vi "NMEA_ParseMessage-WIMDA.vi"(9 "Error In":errorcluster, 10 "$WIMDA-message_IN":string="$WIMDA,29.7101,I,1.0061,B,28.7,C,,,60.8,,20.3,C,,,,,,,,*7B") -> (1 "Error Out":errorcluster, 2 "$WIMDA-message_OUT":T1)   [LabVIEW 2016, in "AIRMAR WeatherCaster.lvlib"]
doc: "<B>GPGGA</B>\nGlobal Positioning System Fix Data"
uses:
  AIRMAR WeatherCaster.lvlib
  NMEA_WIMDA-data.ctl
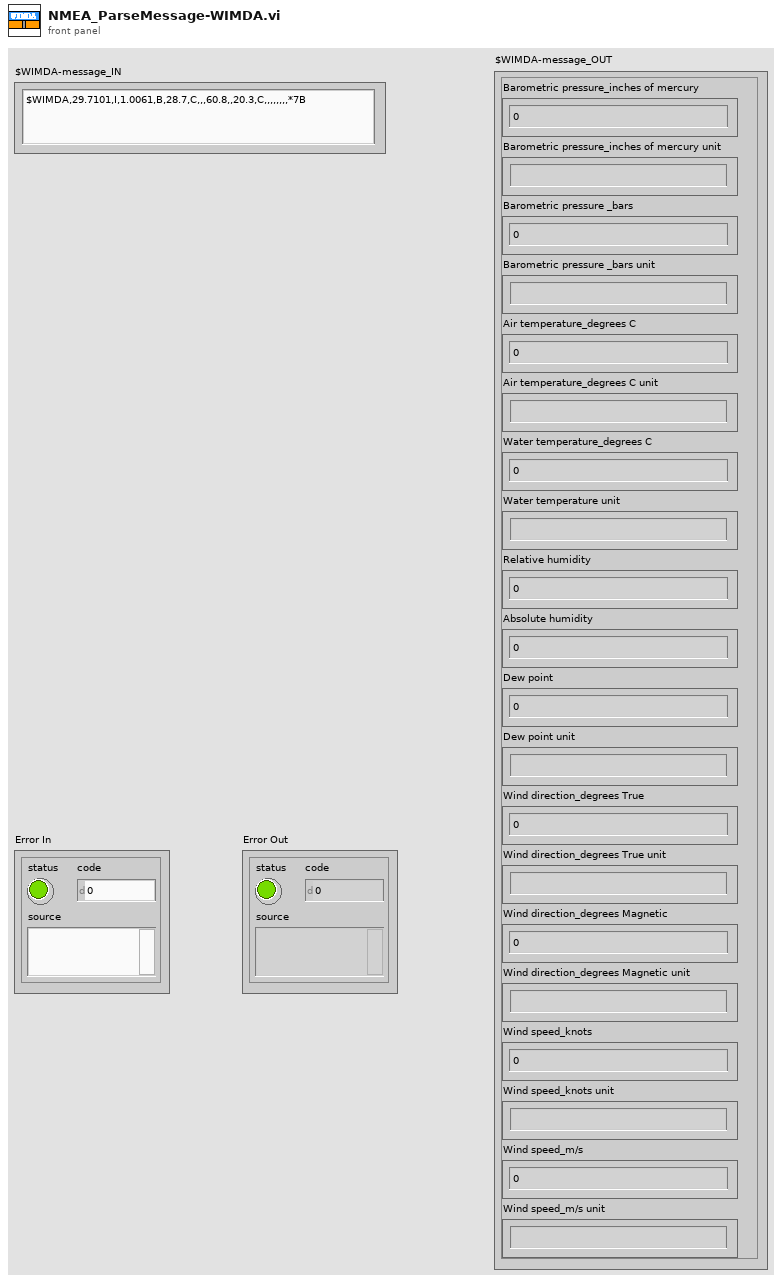
[diagram p1: front panel]
types:
  T1 = typedef "AIRMAR WeatherCaster.lvlib/NMEA_WIMDA-data.ctl" = cluster{"Barometric pressure_inches of mercury":dbl, "Barometric pressure_inches of mercury unit":string, "Barometric pressure _bars":dbl, "Barometric pressure _bars unit":string, "Air temperature_degrees C":dbl, "Air temperature_degrees C unit":string, "Water temperature_degrees C":dbl, "Water temperature unit":string, "Relative humidity":dbl, "Absolute humidity":dbl, "Dew point":dbl, "Dew point unit":string, "Wind direction_degrees True":dbl, "Wind direction_degrees True unit":string, "Wind direction_degrees Magnetic":dbl, "Wind direction_degrees Magnetic unit":string, "Wind speed_knots":dbl, "Wind speed_knots unit":string, "Wind speed_m/s":dbl, "Wind speed_m/s unit":string}
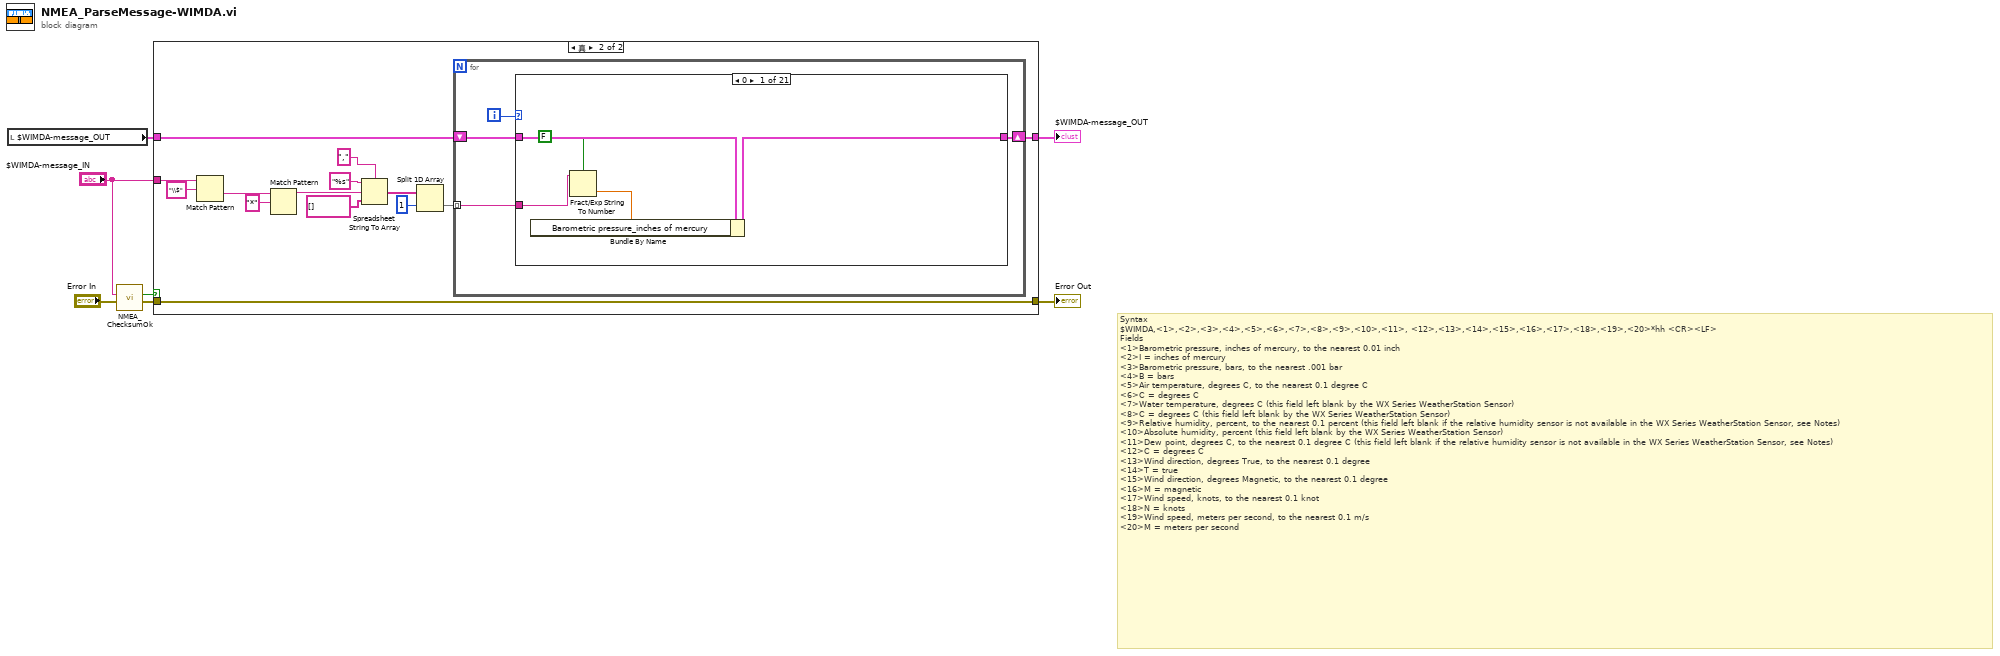
[diagram p0: block diagram]
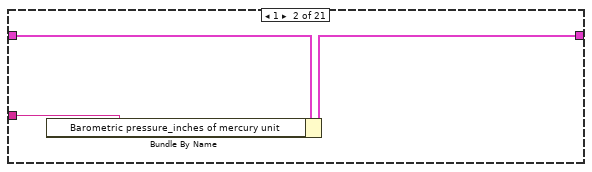
[diagram p3: hidden frame]
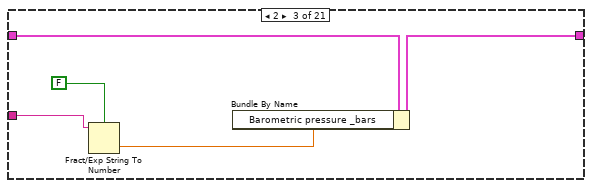
[diagram p4: hidden frame]
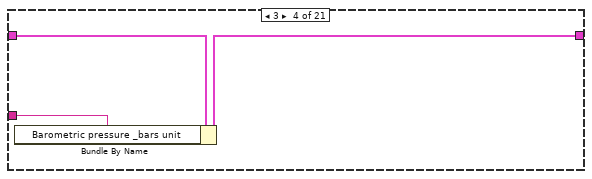
[diagram p5: hidden frame]
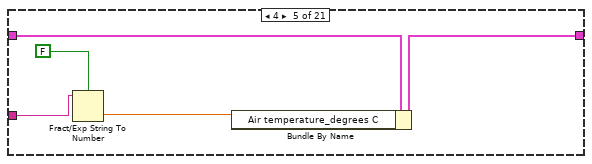
[diagram p6: hidden frame]
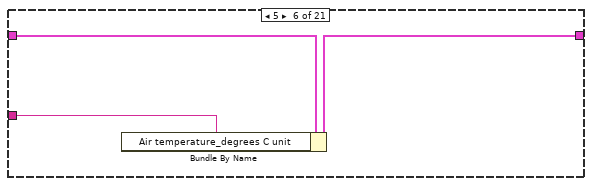
[diagram p7: hidden frame]
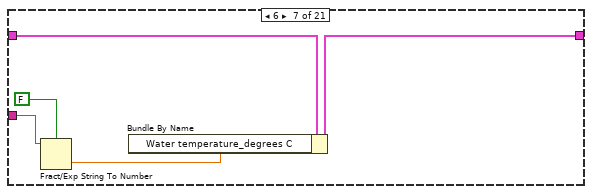
[diagram p8: hidden frame]
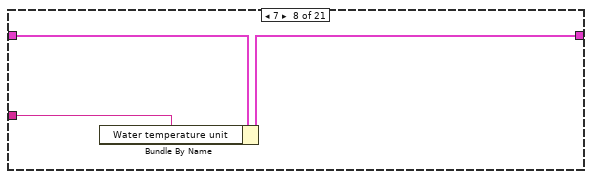
[diagram p9: hidden frame]
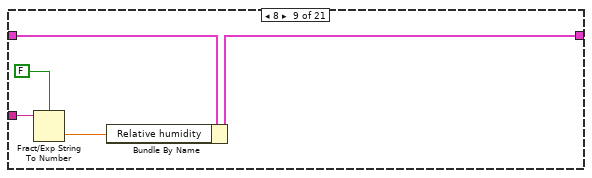
[diagram p10: hidden frame]
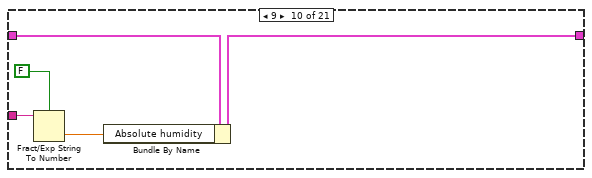
[diagram p11: hidden frame]
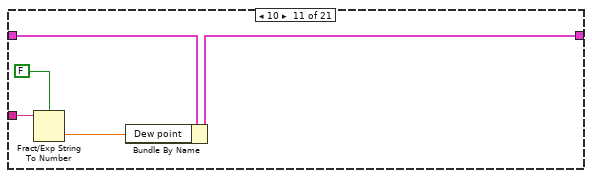
[diagram p12: hidden frame]
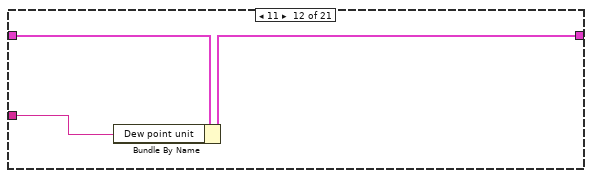
[diagram p13: hidden frame]
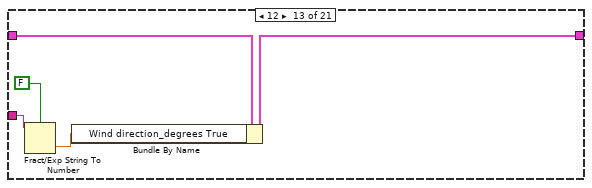
[diagram p14: hidden frame]
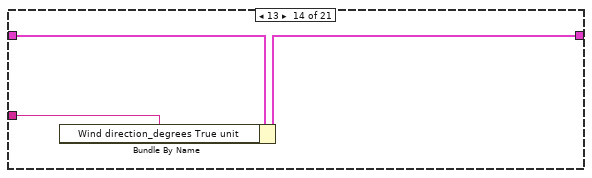
[diagram p15: hidden frame]
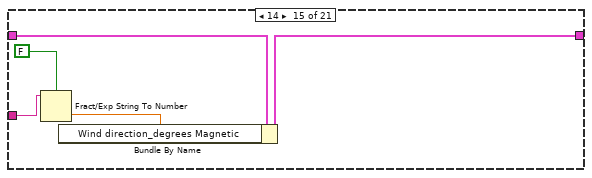
[diagram p16: hidden frame]
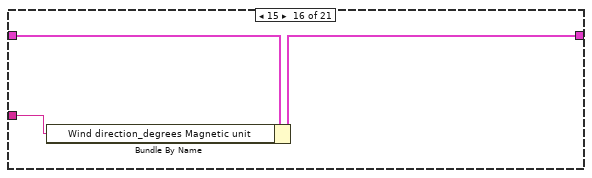
[diagram p17: hidden frame]
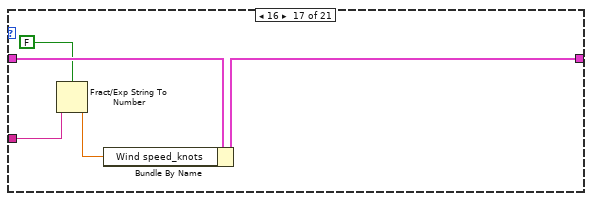
[diagram p18: hidden frame]
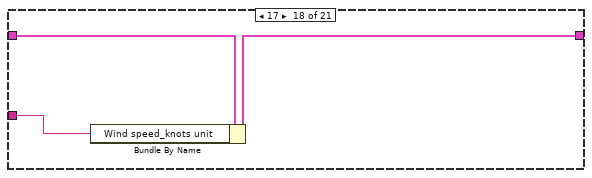
[diagram p19: hidden frame]
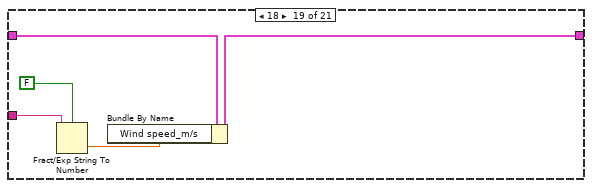
[diagram p20: hidden frame]
diagram:
  # "Syntax\n$WIMDA,<1>,<2>,<3>,<4>,<5>,<6>,<7>,<8>,<9>,<10>,<11>, <12>,<13>,<14>,<15>,<16>,<17>,<18>,<19>,<20>*hh <CR><LF>\nFields\n<1>Barometric pressure, inches of mercury, to the nearest 0.01 inch\n<2>I = inches of mercury\n<3>Barometric pressure, bars, to the nearest .001 bar\n<4>B = bars\n<5>Air temperature, degrees C, to the nearest 0.1 degree C\n<6>C = degrees C\n<7>Water temperature, degrees C (this field left blank by the WX Series WeatherStation Sensor)\n<8>C = degrees C (this field left blank by the WX Series WeatherStation Sensor)\n<9>Relative humidity, percent, to the nearest 0.1 percent (this field left blank if the relative humidity sensor is not available in the WX Series WeatherStation Sensor, see Notes)\n<10>Absolute humidity, percent (this field left blank by the WX Series WeatherStation Sensor)\n<11>Dew point, degrees C, to the nearest 0.1 degree C (this field left blank if the relative humidity sensor is not available in the WX Series WeatherStation Sensor, see Notes)\n<12>C = degrees C\n<13>Wind direction, degrees True, to the nearest 0.1 degree\n<14>T = true\n<15>Wind direction, degrees Magnetic, to the nearest 0.1 degree\n<16>M = magnetic\n<17>Wind speed, knots, to the nearest 0.1 knot\n<18>N = knots\n<19>Wind speed, meters per second, to the nearest 0.1 m/s\n<20>M = meters per second"
  n1 = local read "$WIMDA-message_OUT"() -> (w7:T1)
  n2 = call "NMEA_ChecksumOk.vi"("Error In"="Error In", "Sentence"="$WIMDA-message_IN") -> ("Error Out"=w1:errorcluster, "CheckSumOk?"=w4:bool)  [unwired: 8 in]
  n3 = case shown="真" w4 {
    tunnel: w7 -> [w9 w18]
    tunnel: [w9 w17] -> w6
    tunnel: "$WIMDA-message_IN" -> [_ w15]
    tunnel: w1 -> [w8 w10]
    tunnel: [w8 w10] -> w3
    frame False {
    }
    frame True {
      n4 = Match Pattern(string=w15, regular expression="\\$") -> (after substring=w14:string)  [unwired: 1 in, 3 out]
      n5 = Match Pattern(string=w14, regular expression="*") -> (before substring=w22:string)  [unwired: 1 in, 3 out]
      n6 = Spreadsheet String To Array(delimiter (Tab)=",", format string="%s", spreadsheet string=w22, array type (2D Dbl)=string[] []) -> (array=w12:string[])
      n7 = Split 1D Array(array=w12, index=1) -> (second subarray=w13:string[])  [unwired: 1 out]
      n8 = for {
        tunnel: w13 -> [w24] mode=indexing
        shift-right: [w26] -> w17
        shift-left: w18 -> [w27]
        i -> [w25]
        n9 = case shown="0" w25 {
          tunnel: w27 -> [w32 w35 w40 w43 w48 w50 w56 w59 w64 w69 w74 w77 w82 w85 w90 w93 w98 w101 w106 w109 w110]
          tunnel: [w31 w34 w39 w42 w47 w51 w55 w58 w63 w68 w73 w76 w81 w84 w89 w92 w97 w100 w105 w108 w110] -> w26
          tunnel: w24 -> [w30 w33 w38 w41 w46 w49 w54 w57 w62 w67 w72 w75 w80 w83 w88 w91 w96 w99 w104 w107 _]
          frame 0 {
            n10 = Fract/Exp String To Number(use system decimal point (T)=FALSE ("使用系统小数点(T)"), string=w30) -> (number=w29:dbl)  [unwired: 2 in, 1 out]
            n11 = Bundle By Name(cluster=w32, "Barometric pressure_inches of mercury"=w29) -> (w31:T1)
          }
          frame 1 {
            n12 = Bundle By Name(cluster=w35, "Barometric pressure_inches of mercury unit"=w33) -> (w34:T1)
          }
          frame 2 {
            n13 = Fract/Exp String To Number(use system decimal point (T)=FALSE ("使用系统小数点(T)"), string=w38) -> (number=w36:dbl)  [unwired: 2 in, 1 out]
            n14 = Bundle By Name(cluster=w40, "Barometric pressure _bars"=w36) -> (w39:T1)
          }
          frame 3 {
            n15 = Bundle By Name(cluster=w43, "Barometric pressure _bars unit"=w41) -> (w42:T1)
          }
          frame 4 {
            n16 = Fract/Exp String To Number(use system decimal point (T)=FALSE ("使用系统小数点(T)"), string=w46) -> (number=w44:dbl)  [unwired: 2 in, 1 out]
            n17 = Bundle By Name(cluster=w48, "Air temperature_degrees C"=w44) -> (w47:T1)
          }
          frame 5 {
            n18 = Bundle By Name(cluster=w50, "Air temperature_degrees C unit"=w49) -> (w51:T1)
          }
          frame 6 {
            n19 = Fract/Exp String To Number(use system decimal point (T)=FALSE ("使用系统小数点(T)"), string=w54) -> (number=w52:dbl)  [unwired: 2 in, 1 out]
            n20 = Bundle By Name(cluster=w56, "Water temperature_degrees C"=w52) -> (w55:T1)
          }
          frame 7 {
            n21 = Bundle By Name(cluster=w59, "Water temperature unit"=w57) -> (w58:T1)
          }
          frame 8 {
            n22 = Fract/Exp String To Number(use system decimal point (T)=FALSE ("使用系统小数点(T)"), string=w62) -> (number=w61:dbl)  [unwired: 2 in, 1 out]
            n23 = Bundle By Name(cluster=w64, "Relative humidity"=w61) -> (w63:T1)
          }
          frame 9 {
            n24 = Fract/Exp String To Number(use system decimal point (T)=FALSE ("使用系统小数点(T)"), string=w67) -> (number=w66:dbl)  [unwired: 2 in, 1 out]
            n25 = Bundle By Name(cluster=w69, "Absolute humidity"=w66) -> (w68:T1)
          }
          frame 10 {
            n26 = Fract/Exp String To Number(use system decimal point (T)=FALSE ("使用系统小数点(T)"), string=w72) -> (number=w71:dbl)  [unwired: 2 in, 1 out]
            n27 = Bundle By Name(cluster=w74, "Dew point"=w71) -> (w73:T1)
          }
          frame 11 {
            n28 = Bundle By Name(cluster=w77, "Dew point unit"=w75) -> (w76:T1)
          }
          frame 12 {
            n29 = Fract/Exp String To Number(use system decimal point (T)=FALSE ("使用系统小数点(T)"), string=w80) -> (number=w79:dbl)  [unwired: 2 in, 1 out]
            n30 = Bundle By Name(cluster=w82, "Wind direction_degrees True"=w79) -> (w81:T1)
          }
          frame 13 {
            n31 = Bundle By Name(cluster=w85, "Wind direction_degrees True unit"=w83) -> (w84:T1)
          }
          frame 14 {
            n32 = Fract/Exp String To Number(use system decimal point (T)=FALSE ("使用系统小数点(T)"), string=w88) -> (number=w87:dbl)  [unwired: 2 in, 1 out]
            n33 = Bundle By Name(cluster=w90, "Wind direction_degrees Magnetic"=w87) -> (w89:T1)
          }
          frame 15 {
            n34 = Bundle By Name(cluster=w93, "Wind direction_degrees Magnetic unit"=w91) -> (w92:T1)
          }
          frame 16 {
            n35 = Fract/Exp String To Number(use system decimal point (T)=FALSE ("使用系统小数点(T)"), string=w96) -> (number=w94:dbl)  [unwired: 2 in, 1 out]
            n36 = Bundle By Name(cluster=w98, "Wind speed_knots"=w94) -> (w97:T1)
          }
          frame 17 {
            n37 = Bundle By Name(cluster=w101, "Wind speed_knots unit"=w99) -> (w100:T1)
          }
          frame 18 {
            n38 = Fract/Exp String To Number(use system decimal point (T)=FALSE ("使用系统小数点(T)"), string=w104) -> (number=w103:dbl)  [unwired: 2 in, 1 out]
            n39 = Bundle By Name(cluster=w106, "Wind speed_m/s"=w103) -> (w105:T1)
          }
          frame 19 {
            n40 = Bundle By Name(cluster=w109, "Wind speed_m/s unit"=w107) -> (w108:T1)
          }
          frame Default {
          }
        }
      }
    }
  }
  "$WIMDA-message_OUT" <- w6
  "Error Out" <- w3
